vi "MFC W REG reset.vi"   [LabVIEW 2011]
uses:
  <vilib>/rvi/eio/common/nirviEmuTemplateMethod_errors.vi
  <vilib>/eio/EIOMethodNode/EIOMethodNode.xnode
panel:
  # "this VI set to default the gas MFCs"
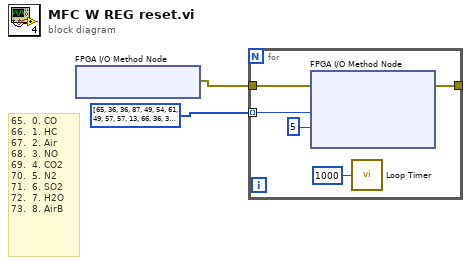
[diagram p0: block diagram]
diagram:
  # "65.  0. CO\n66.  1. HC\n67.  2. Air\n68.  3. NO\n69.  4. CO2\n70.  5. N2\n71.  6. SO2\n72.  7. H2O\n73.  8. AirB"
  n1 = xnode "FPGA I/O Method Node"() -> ("error out"=w2:errorcluster)  [unwired: 2 in, 1 out]
  n2 = for {
    tunnel: i16[] [65, 36, 36, 87, 49, 54, 61, 49, 57, 57, 13, 66, 36, 36, 87, 49, 54, 61, 49, 57, 57, 13, 67, 36, 36, 87, 49, 54, 61, 49, 57, 57, 13, 68, 36, 36, 87, 49, 54, 61, 49, 57, 57, 13, 69, 36, 36, 87, 49, 54, 61, 49, 57, 57, 13, 70, 36, 36, 87, 49, 54, 61, 49, 57, 57, 13, 71, 36, 36, 87, 49, 54, 61, 49, 57, 57, 13, 72, 36, 36, 87, 49, 54, 61, 51, 56, 13, 73, 36, 36, 87, 49, 54, 61, 49, 57, 57, 13] ("Array 3") -> [w6] mode=indexing
    tunnel: [w4] -> _
    tunnel: w2 -> [w3]
    n3 = xnode "FPGA I/O Method Node"("error in"=w3, "Data"=w6, "Timeout (ms)"=5) -> ("error out"=w4:errorcluster)  [unwired: 1 in, 2 out]
    n4 = call "Loop Timer"("Count(uSec)"=u32 1000) -> ()  [unwired: 1 out]
  }
